vi "Wait For Task_core.vi"(8 "error in (no error)":errorcluster, 11 "HttpResponseMessage in":refnum<class "HttpResponseMessage.lvclass">) -> (0 "error out":errorcluster, 1 "IsCompleted":bool, 3 "HttpResponseMessage out":refnum<class "HttpResponseMessage.lvclass">, 4 "Timeout":bool)   [LabVIEW 2018, in "HttpClient_NET.lvlib" / "HttpResponseMessage.lvclass"]
uses:
  HttpResponseMessage.lvclass
  HttpResponseMessage.lvclass/HttpResponseMessage.ctl
  Accessors/Read NET_HttpResponseTask.vi
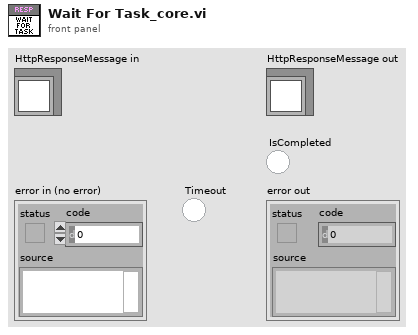
[diagram p1: front panel]
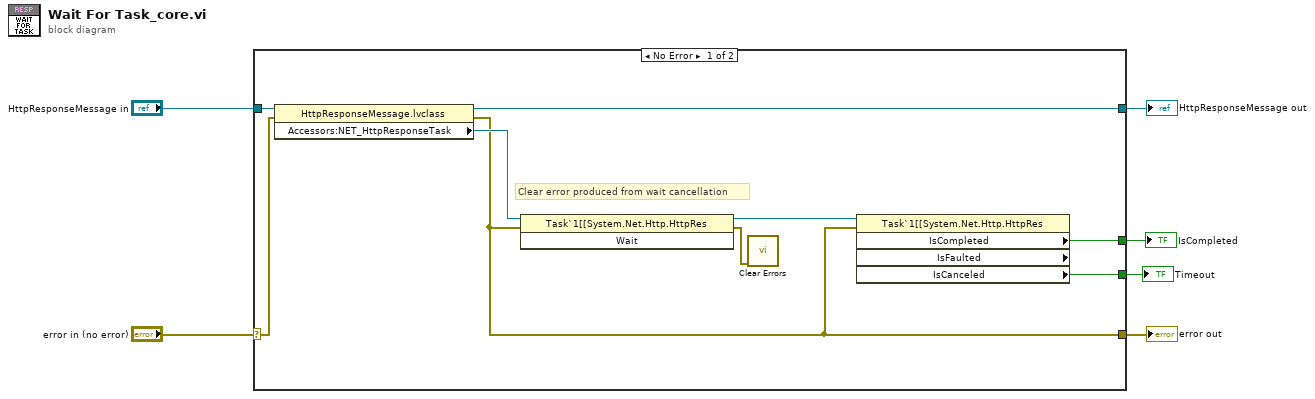
[diagram p0: block diagram]
diagram:
  n1 = case shown="No Error" "error in (no error)" {
    selector: "error in (no error)" -> [w15 w17]
    tunnel: [w8 w17] -> w5
    tunnel: [w13 w16] -> w3
    tunnel: "HttpResponseMessage in" -> [w14 w16]
    tunnel: [w11 _] -> w2
    tunnel: [w10 _] -> w1
    frame No Error {
      # "Clear error produced from wait cancellation"
      n2 = property class="HttpResponseMessage.lvclass"(reference=w14, error in=w15) -> (reference out=w13:refnum<class "HttpResponseMessage.lvclass">, error out=w8:errorcluster, "Accessors:NET_HttpResponseTask"=w12:refnum<k24>)
      n3 = invoke class="Task`1[[System.Net.Http.HttpRes" method="Wait"(reference=w12, error in=w8) -> (reference out=w9:refnum<k24>, error out=w7:errorcluster)  [unwired: 1 in, 1 out]
      n4 = call <vilib>:"Clear Errors.vi"("error in (no error)"=w7) -> ()  [unwired: 5 in, 2 out]
      n5 = property class="Task`1[[System.Net.Http.HttpRes" props=["IsCompleted", "IsFaulted", "IsCanceled"](reference=w9, error in=w8) -> ("IsCompleted"=w11:bool, "IsCanceled"=w10:bool)  [unwired: 3 out]
    }
    frame Error {
    }
  }
  "error out" <- w5
  "HttpResponseMessage out" <- w3
  "IsCompleted" <- w2
  "Timeout" <- w1
